vi "SolidTargetSequenceControl.vi"() -> ()   [LabVIEW 2015]
uses:
  ShootingStar/ShootingStar.lvlib
  State.ctl
  SolidTargetSequenceControl.lvlib
  <vilib>/Instr/_visa.llb/VISA Configure Serial Port (Instr).vi
  NetworkStream/NetworkStreamReceiverState.ctl
  NetworkStream/NetworkStream.lvlib
  NetworkStream/NetworkStreamData.ctl
  <vilib>/dex/Stream Element Allocation Mode.ctl
  NetworkStream/NetworkStreamReceiverMainQueueCluster.ctl
  NetworkStream/NetworkStreamStateMachineVariable.ctl
  NetworkStream/NetworkStreamReceiverStatusEventCluster.ctl
  ConsumerLoopVariable.ctl
  <vilib>/Utility/error.llb/Error Cluster From Error Code.vi
  <vilib>/ErrorRing/Error Ring.xnode
panel:
  in  "Arduino Serial Port":refnum<visa-resource-name>="COM3"
  in  "Phidget Voltage (V)":dbl=2.0 min=-10.0 max=10.0 step=0.1
  out "Device State":T1
  out "Session Hash":u64
  out "Network Stream State Indicator":T2
  in  "Shoot Once":bool
  in  "Target Radius (mm)":dbl=50.6
  in  "Shooting Pos. (mm)":dbl=5.0
  in  "Acquisition Time (ms)":dbl=100.0
  in  "Shot Spacing (mm)":dbl=0.1
  in  "Target Edge Pos. (mm)":dbl
  in  "Stop Rotation":bool
  in  "Start Rotation":bool
  in  "Clear Phidget":bool
  in  "Trig Cam":bool
  out "Arduino Message":string
  in  "Clear Serial Error":bool
  out "Phidget Error Cluster":errorcluster
  out "Cible":cluster{dbl, dbl}(knob)={0.0, 5.935711578539576} scale=0.0..360.0
  out "SP RotatingSpeed \n(deg/s)":dbl
  out "SP RotatingSpeed \n(rad/s)":dbl
  out "Serial error":errorcluster caption="Serial Error Out"
  in  "Calibrate":bool
  in  "ResetShotUntil":bool
  out "Shot until (°)":dbl
  out "Target position (°)":dbl
  in  "stop":bool
  # "Target Settings"
  # "Target Rotation"
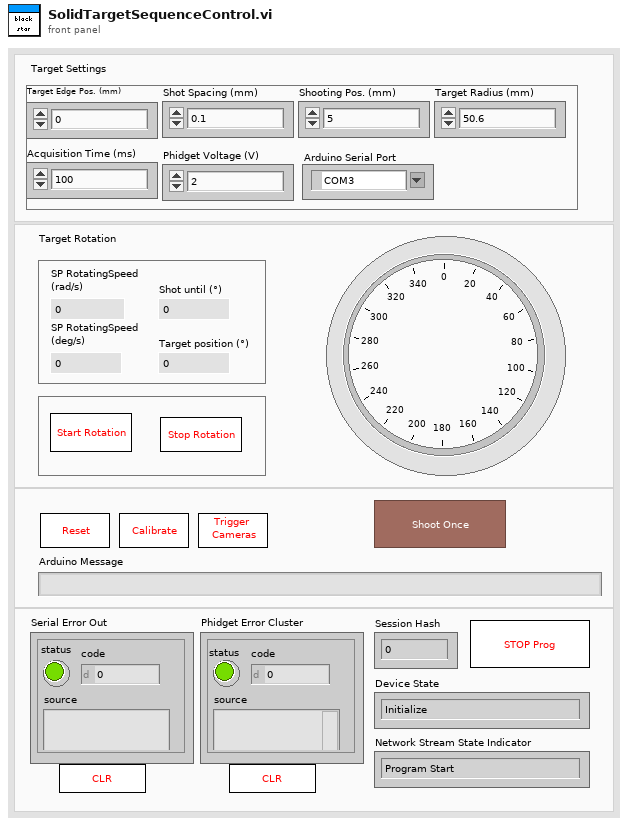
[diagram p1: front panel]
types:
  T1 = typedef "SolidTargetSequenceControl.lvlib/State.ctl" = enum16{"Initialize", "Running", "Closing"}
  T2 = typedef "NetworkStream.lvlib/NetworkStreamReceiverState.ctl" = enum16{"Program Start", "Waiting for connection", "Connected", "Connection lost", "Exit", "Unhandled Exception"}
  T3 = typedef "SolidTargetSequenceControl.lvlib/ConsumerLoopVariable.ctl" = cluster{"Arduino Serial Port":refnum<visa-resource-name>, "Phidget device handle":i32, "Arduino Message":string, "TargetRotating":bool}
  T4 = typedef "NetworkStream.lvlib/NetworkStreamReceiverStatusEventCluster.ctl" = cluster{"Status":string, "Data":variant, "SequenceNumber":u64}
  T5 = typedef "NetworkStream.lvlib/NetworkStreamStateMachineVariable.ctl" = cluster{"Network Stream Reader Endpoint":refnum<k21>, "Last Received Sequence Number":u64}
  T6 = typedef "NetworkStream.lvlib/NetworkStreamReceiverMainQueueCluster.ctl" = cluster{"Command":string, "Data":variant, "SequenceNumber":u64}
  T7 = enum8{"Enabled", "Disabled", "Disabled and Grayed Out"}
  T8 = typedef "NetworkStream.lvlib/NetworkStreamData.ctl" = cluster{"Command/Status":string, "Data":variant, "Session Hash":u64, "Sequence Number":u64}
  T9 = typedef "Stream Element Allocation Mode.ctl" = u32
  T10 = cluster{"Command/Status":string, "Data":variant, "Sequence Number":u64}
  T11 = cluster{"Status":string, "Data":variant, "Session Hash":u64, "SequenceNumberOfFinishedCommand":u64}
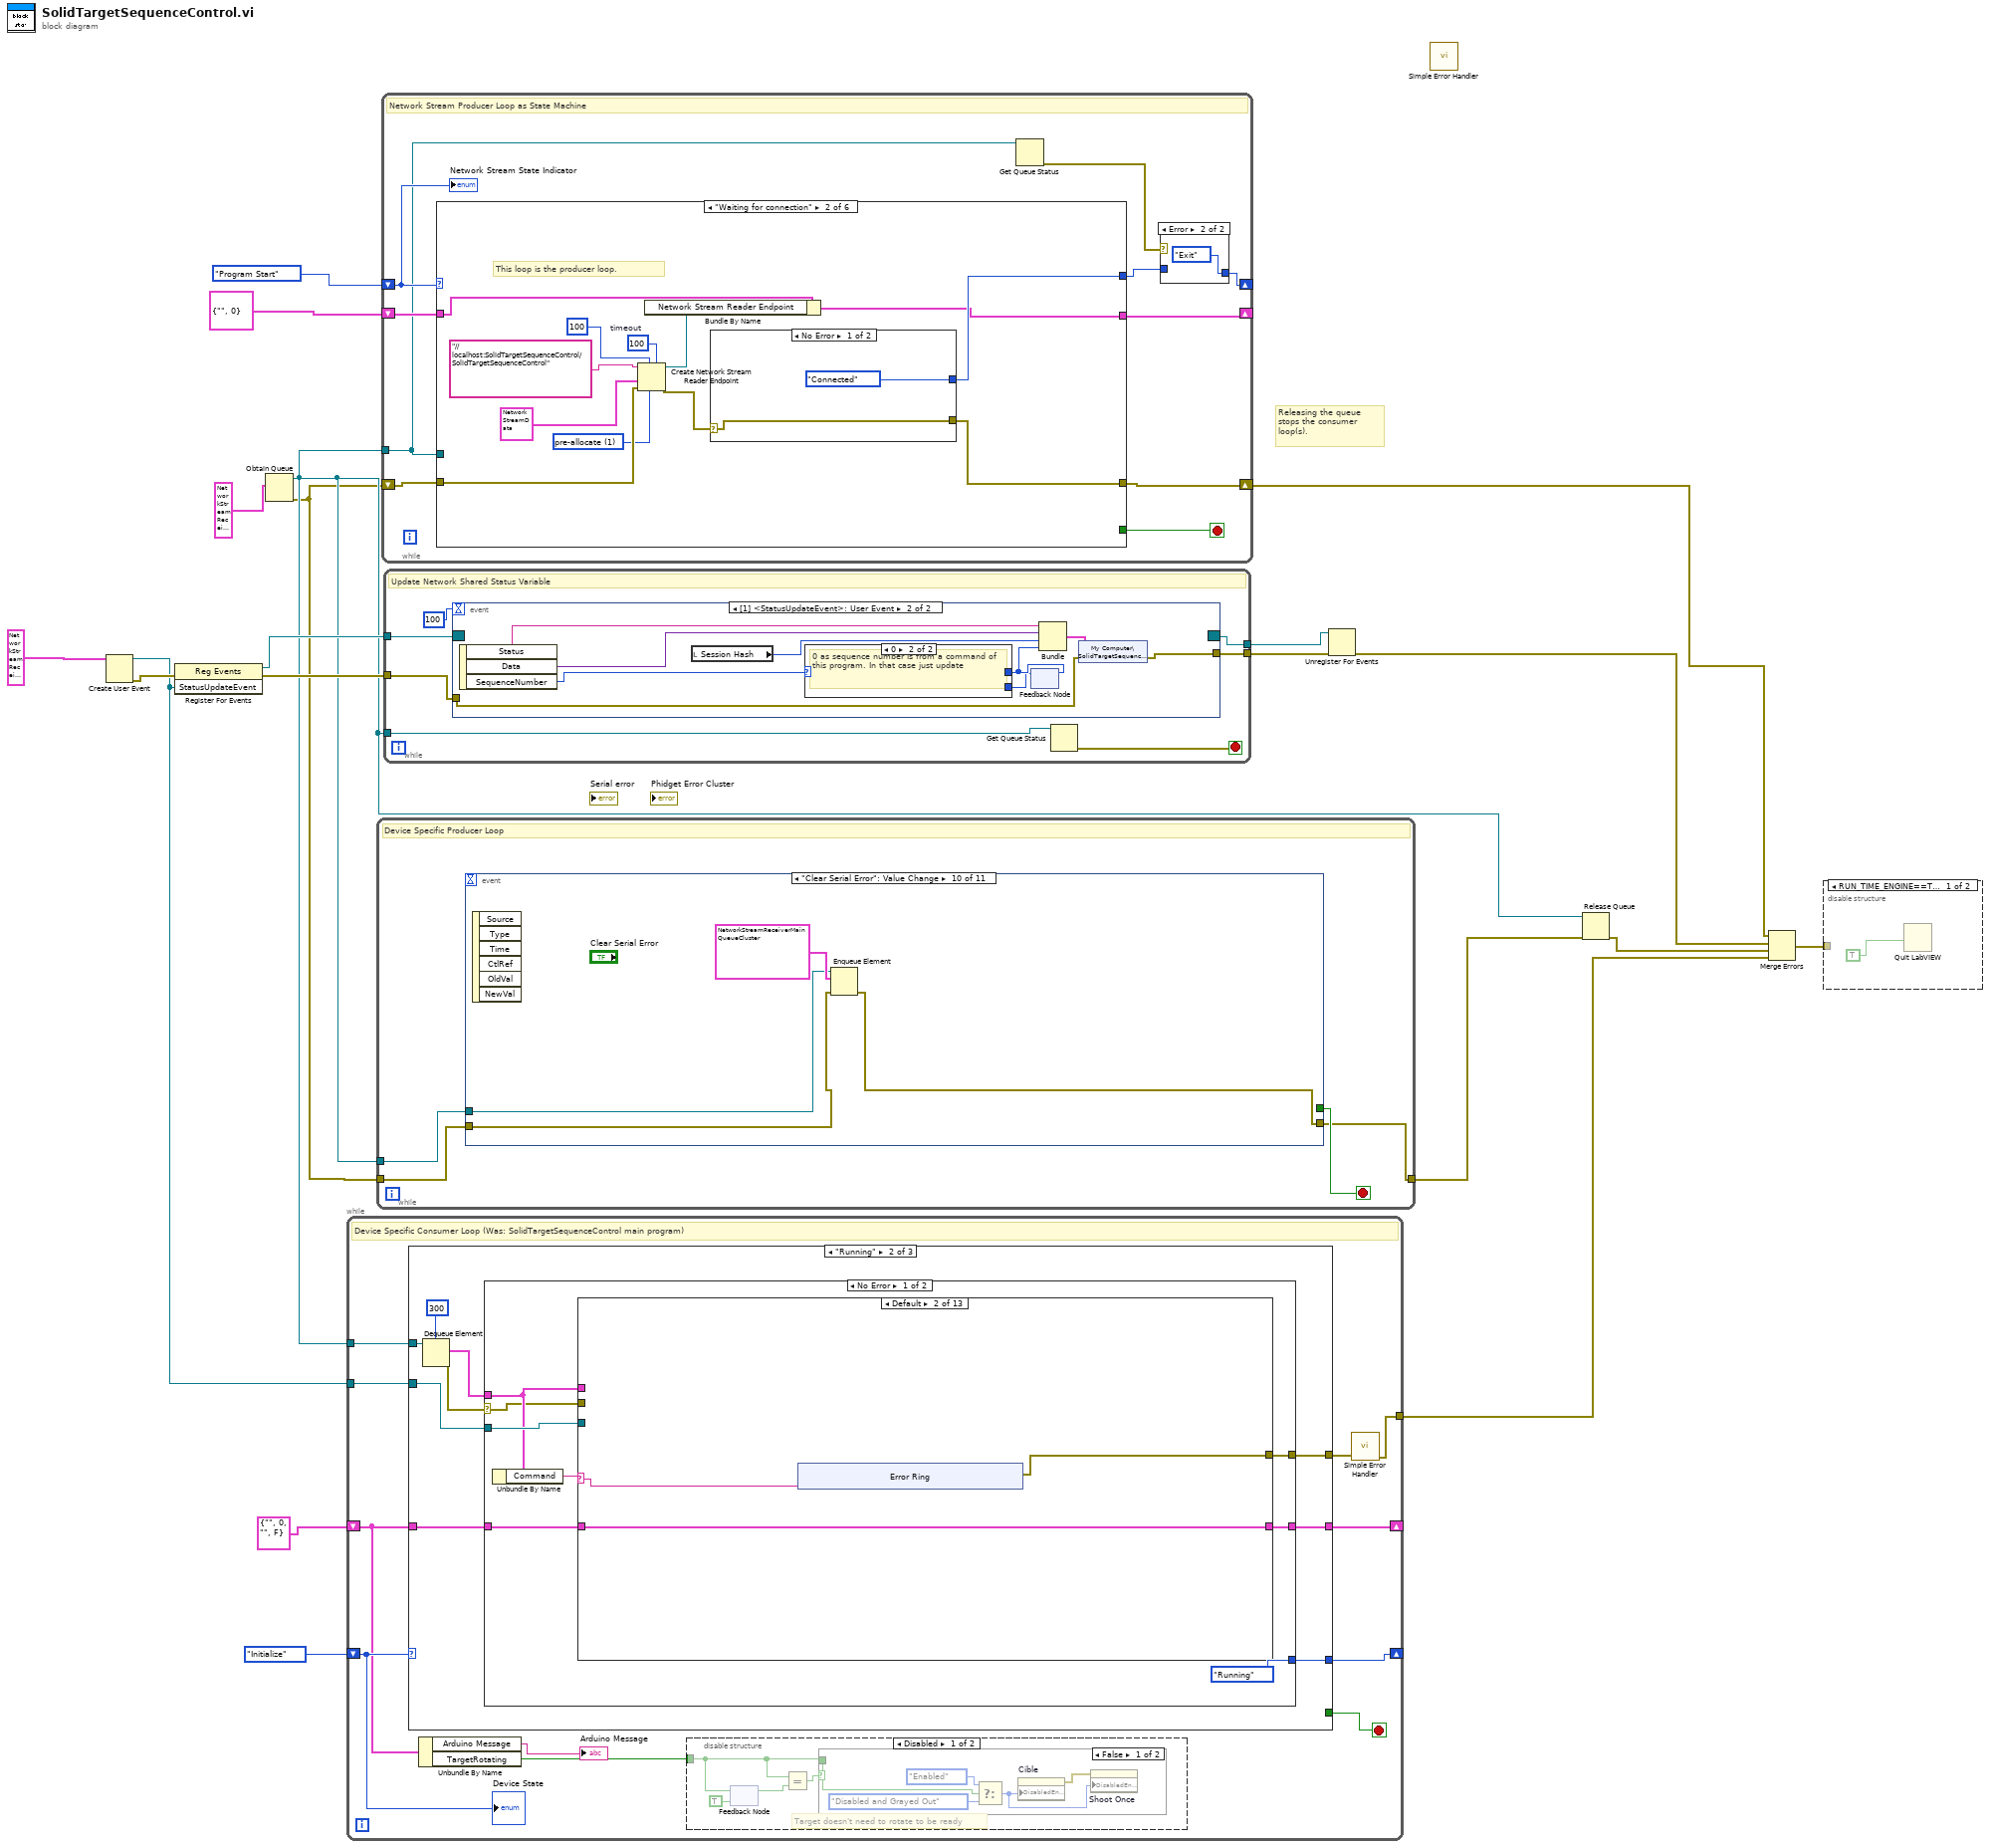
[diagram p0: block diagram]
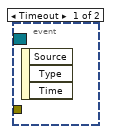
[diagram p2: hidden frame]
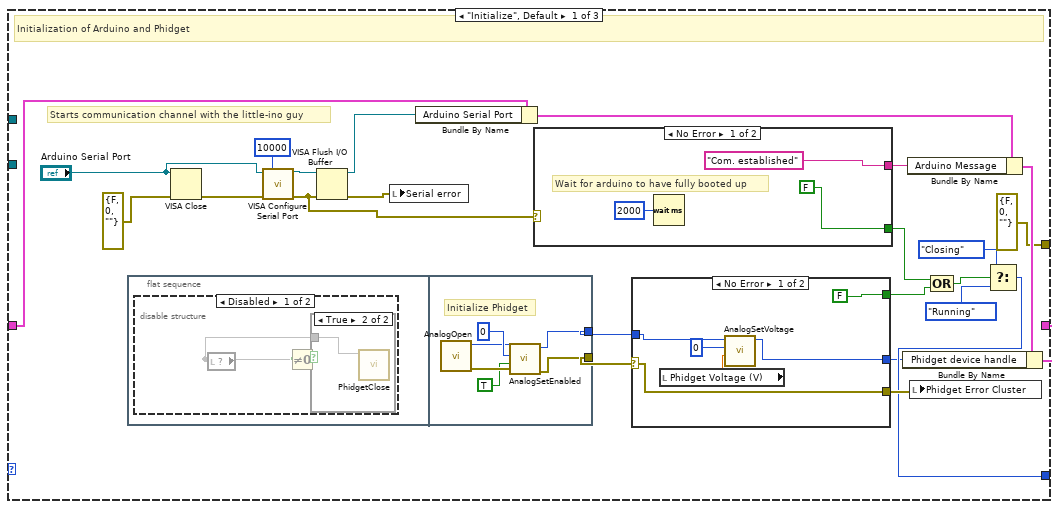
[diagram p6: hidden frame]
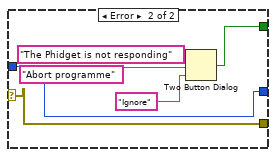
[diagram p7: hidden frame]
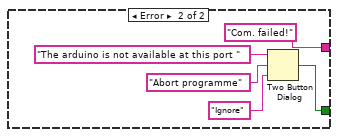
[diagram p10: hidden frame]
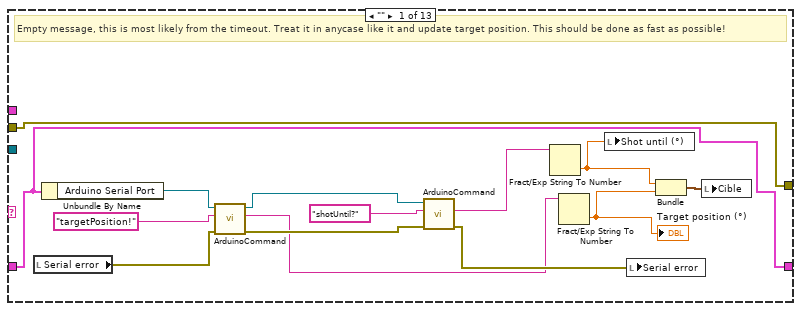
[diagram p11: hidden frame]
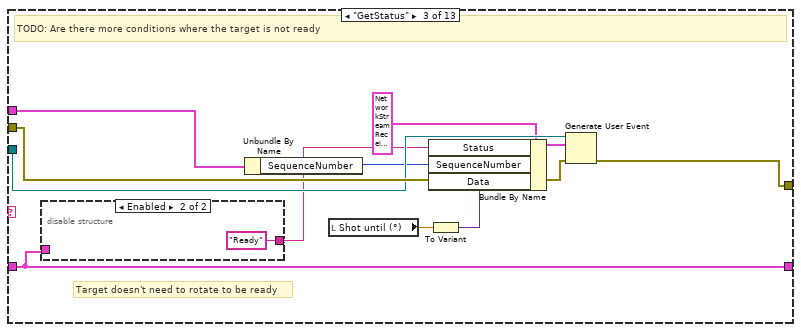
[diagram p12: hidden frame]
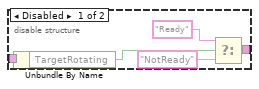
[diagram p13: hidden frame]
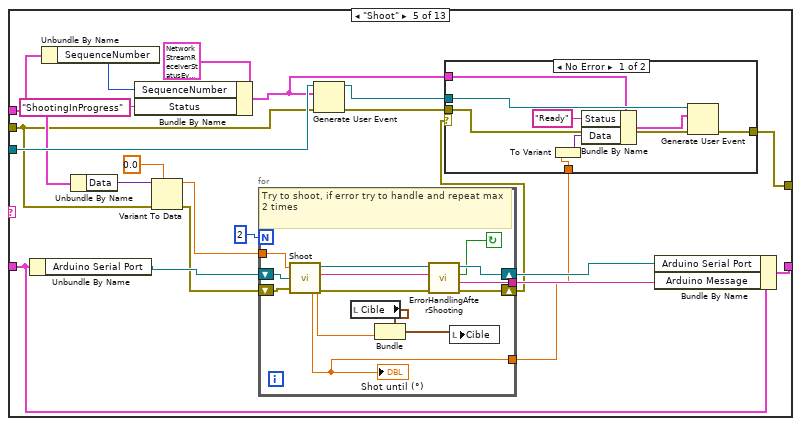
[diagram p15: hidden frame]
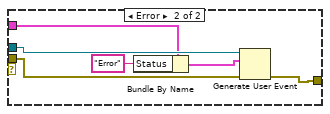
[diagram p16: hidden frame]
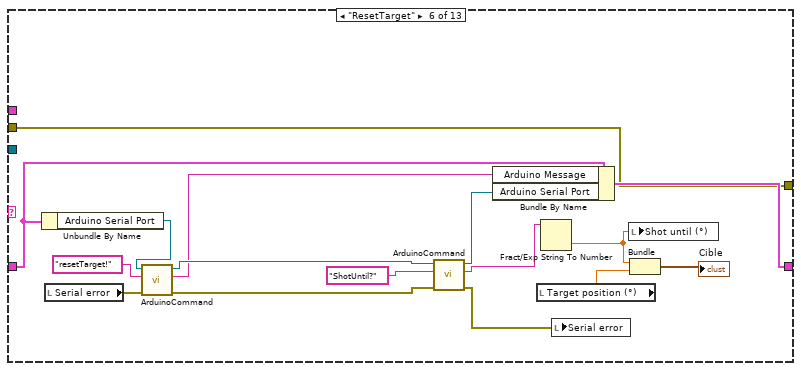
[diagram p17: hidden frame]
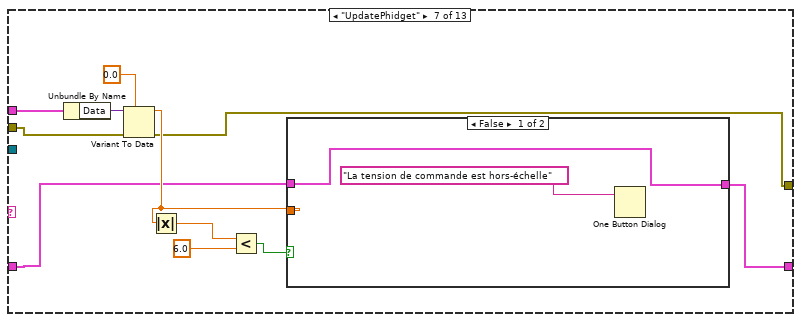
[diagram p18: hidden frame]
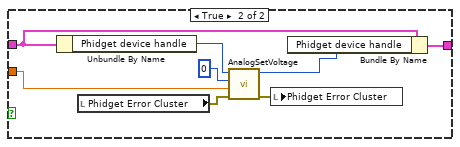
[diagram p19: hidden frame]
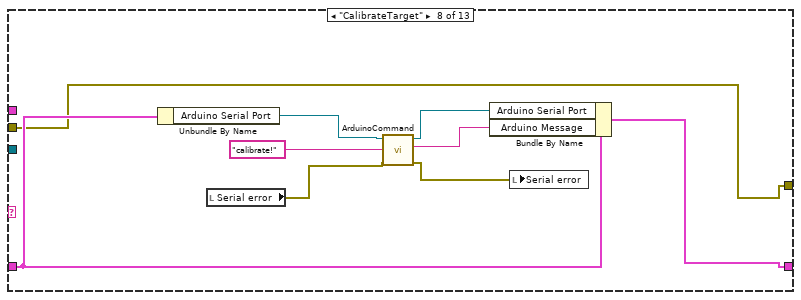
[diagram p20: hidden frame]
diagram:
  # "Releasing the queue stops the consumer loop(s)."
  n1 = Create User Event(user event datatype=T4 {"Status"="", "Data"=variant, "SequenceNumber"=0} ("StatusUpdateEvent")) -> (user event=w11:refnum<user-event>, error out=w17:errorcluster)  [unwired: 1 in]
  n2 = register-events(error in=w17, w11) -> (reference out=w16:refnum<event-registration>, error out=w13:errorcluster)  [unwired: 1 in]
  n3 = Obtain Queue(element data type=T6 {"Command"="", "Data"=variant, "SequenceNumber"=0}) -> (queue out=w10:refnum<queue>, error out=w9:errorcluster)  [unwired: 4 in, 1 out]
  n4 = while {
    tunnel: w10 -> [w31]
    tunnel: w11 -> [w29]
    tunnel: [w22] -> w3
    shift-right: [w27] -> _
    shift-left: State."Initialize" -> [w28]
    shift-right: [w26] -> _
    shift-left: T3 {"Arduino Serial Port"="", "Phidget device handle"=0, "Arduino Message"="", "TargetRotating"=FALSE} ("Cluster") -> [w24]
    stop <- w30 stop-if-true
    # "Device Specific Consumer Loop (Was: SolidTargetSequenceControl main program)"
    n5 = case shown="\"Running\"" w28 {
      tunnel: w31 -> [_ w102 _]
      tunnel: [_ _ TRUE] -> w30
      tunnel: w29 -> [_ w99 _]
      tunnel: [w50 w98 State."Initialize"] -> w27
      tunnel: w24 -> [w48 w96 w319]
      tunnel: [w45 w95 T3 {"Arduino Serial Port"="", "Phidget device handle"=0, "Arduino Message"="Connection Closed", "TargetRotating"=FALSE} ("Cluster")] -> w26
      tunnel: [errorcluster {"status"=FALSE, "code"=0, "source"=""} ("error out") w97 errorcluster {"status"=FALSE, "code"=0, "source"=""} ("error out")] -> w23
      frame "Initialize", Default {
        # "Starts communication channel with the little-ino guy"
        # "Initialization of Arduino and Phidget"
        n6 = flat-sequence {
          tunnel: [w81] -> w61
          tunnel: [w80] -> w62
          frame #0 {
            n7 = disable-structure shown="Disabled" {
              frame Disabled {
                n8 = local read item#-1() -> (w77)
                n9 = Not Equal To 0?(x=w77) -> (x != 0?=w78:bool)
                n10 = case shown="True" w78 {
                  tunnel: w77 -> [_ w79]
                  frame False {
                  }
                  frame True {
                    n11 = call "PhidgetClose.vi"("Device In"=w79) -> ()  [unwired: 10 in, 1 out]
                  }
                }
              }
              frame Enabled {
              }
            }
          }
          frame #1 {
            # "Initialize Phidget"
            n12 = call "AnalogOpen.vi"() -> ("error out"=w85:errorcluster, "Device Out"=w82:i32)  [unwired: 8 in, 2 out]
            n13 = call "AnalogSetEnabled.vi"("error in (no error)"=w85, "SetEnabled"=TRUE, "index"=0, "Device In"=w82) -> ("error out"=w80:errorcluster, "Device Out"=w81:i32)  [unwired: 5 in]
          }
        }
        n14 = VISA Close(VISA resource name="Arduino Serial Port", error in (no error)=errorcluster {"status"=FALSE, "code"=0, "source"=""}) -> (error out=w57:errorcluster)
        n15 = call-poly "VISA Configure Serial Port"("VISA resource name"="Arduino Serial Port", "timeout (10sec)"=u32 10000, "error in (no error)"=w57) -> ("VISA resource name out"=w58:refnum<visa-resource-name>, "error out"=w60:errorcluster)  [unwired: 11 in]
        n16 = VISA Flush I/O Buffer(VISA resource name=w58, error in (no error)=w60) -> (VISA resource name out=w47:refnum<visa-resource-name>, error out=w55:errorcluster)  [unwired: 1 in]
        n17 = local write "Serial error"(w55) -> ()
        n18 = Bundle By Name(cluster=w48, "Arduino Serial Port"=w47) -> (w44:T3)
        n19 = case shown="No Error" w60 {
          tunnel: [FALSE ("T button?") w92] -> w53
          tunnel: ["Com. established" ("Arduino Message") "Com. failed!" ("Arduino Message")] -> w42
          frame No Error {
            # "Wait for arduino to have fully booted up"
            n20 = Wait (ms)(milliseconds to wait=u32 2000) -> ()  [unwired: 1 out]
          }
          frame Error {
            n21 = Two Button Dialog(message="The arduino is not available at this port ", 1:"Ignore" ("Nom du bouton V (\"OK\")"), 2:"Abort programme" ("Nom du bouton V (\"OK\")")) -> (T button?=w92:bool)
          }
        }
        n22 = case shown="No Error" w62 {
          selector: w62 -> [w66 w72]
          tunnel: [FALSE w73] -> w54
          tunnel: w61 -> [w69 w71]
          tunnel: [w66 w72] -> w59
          tunnel: [w65 w71] -> w46
          frame No Error {
            n23 = local read "Phidget Voltage (V)"() -> (w67:dbl)
            n24 = call "AnalogSetVoltage.vi"("voltage"=w67, "index"=0, "Device In"=w69) -> ("Device Out"=w65:i32)  [unwired: 6 in, 1 out]
          }
          frame Error {
            n25 = Two Button Dialog(message="The Phidget is not responding", 1:"Ignore" ("Nom du bouton V (\"OK\")"), 2:"Abort programme" ("Nom du bouton V (\"OK\")")) -> (T button?=w73:bool)
          }
        }
        n26 = Bundle By Name(cluster=w44, "Arduino Message"=w42) -> (w43:T3)
        n27 = Bundle By Name(cluster=w43, "Phidget device handle"=w46) -> (w45:T3)
        n28 = local write "Phidget Error Cluster"(w59) -> ()
        n29 = Compound Arithmetic op=OR(w53, w54) -> (w52:bool)
        n30 = Select(t=State."Closing", s=w52, f=State."Running") -> (s? t:f=w50:T1)
      }
      frame "Running" {
        n31 = Dequeue Element(queue=w102, timeout in ms (-1)=300) -> (element=w100:T6, error out=w101:errorcluster)  [unwired: 1 in, 2 out]
        n32 = case shown="No Error" w101 {
          selector: w101 -> [w106 w313]
          tunnel: w100 -> [w108 _]
          tunnel: w99 -> [w110 _]
          tunnel: [State."Running" w314] -> w98
          tunnel: [w105 w312] -> w97
          tunnel: w96 -> [w104 w310]
          tunnel: [w103 w309] -> w95
          frame No Error {
            n33 = Unbundle By Name(w108) -> ("Command"=w109:string)
            n34 = case shown="Default" w109 {
              selector: w109 -> [_ w127 _ _ _ _ _ _ _ _ _ _ _]
              tunnel: w110 -> [_ _ w144 _ w175 _ _ _ _ _ _ _ _]
              tunnel: w108 -> [_ _ w141 _ w170 _ w226 _ _ _ _ _ _]
              tunnel: w106 -> [w111 _ w145 w152 w166 w204 w222 w242 w249 w260 w274 w280 w302]
              tunnel: [w111 w126 w139 w152 w156 w204 w221 w242 w249 w260 w274 w280 w302] -> w105
              tunnel: w104 -> [w112 w125 w138 w153 w163 w207 w220 w244 w254 w262 w276 w283 w304]
              tunnel: [w112 w125 w138 w153 w164 w205 w219 w243 w250 w261 w275 w281 w303] -> w103
              frame "" {
                # "Empty message, this is most likely from the timeout. Treat it in anycase like it and update target position. This should be done as fast as possible!"
                n35 = local read "Serial error"() -> (w118:errorcluster)
                n36 = Unbundle By Name(w112) -> ("Arduino Serial Port"=w113:refnum<visa-resource-name>)
                n37 = call "ArduinoCommand.vi"("entrée d'erreur (pas d'erreur)"=w118, "buffer à écrire"="targetPosition!", "Refnum VISA en entrée"=w113) -> ("sortie d'erreur"=w121:errorcluster, "read buffer"=w117:string, "Refnum VISA en sortie"=w119:refnum<visa-resource-name>)  [unwired: 6 in]
                n38 = call "ArduinoCommand.vi"("entrée d'erreur (pas d'erreur)"=w121, "buffer à écrire"="shotUntil?", "Refnum VISA en entrée"=w119) -> ("sortie d'erreur"=w122:errorcluster, "read buffer"=w123:string)  [unwired: 6 in, 1 out]
                n39 = Fract/Exp String To Number(string=w123) -> (number=w115:dbl)  [unwired: 3 in, 1 out]
                n40 = Fract/Exp String To Number(string=w117) -> (number=w124:dbl)  [unwired: 3 in, 1 out]
                "Target position (°)" <- w124
                n41 = local write "Shot until (°)"(w115) -> ()
                n42 = local write "Serial error"(w122) -> ()
                n43 = Bundle(w115, w124) -> (w114:cluster{dbl, dbl})  [unwired: 1 in]
                n44 = local write "Cible"(w114) -> ()
              }
              frame Default {
                n45 = xnode "Error Ring"("parameter 0"=w127) -> ("error out"=w126:errorcluster)
              }
              frame "GetStatus" {
                # "Target doesn't need to rotate to be ready"
                # "TODO: Are there more conditions where the target is not ready"
                n46 = disable-structure shown="Enabled" {
                  disable-tunnel: w138 -> [w150 _]
                  disable-tunnel: [w147 "Ready" ("f")] -> w137
                  frame Disabled {
                    n47 = Unbundle By Name(w150) -> ("TargetRotating"=w148:bool)
                    n48 = Select(t="Ready" ("Status"), s=w148, f="NotReady") -> (s? t:f=w147:string)
                  }
                  frame Enabled {
                  }
                }
                n49 = Unbundle By Name(w141) -> ("SequenceNumber"=w140:u64)
                n50 = local read "Shot until (°)"() -> (w135:dbl)
                n51 = To Variant(anything=w135) -> (Variant=w136:variant)
                n52 = Bundle By Name(cluster=T4 {"Status"="", "Data"=variant, "SequenceNumber"=0} ("event data"), "Status"=w137, "SequenceNumber"=w140, "Data"=w136) -> (w142:T4)
                n53 = Generate User Event(user event=w144, event data cluster=w142, error in=w145) -> (error out=w139:errorcluster)  [unwired: 1 in, 1 out]
              }
              frame "Reinitialize" {
                # "Todo: Implement"
              }
              frame "Shoot" {
                n54 = Unbundle By Name(w163) -> ("Arduino Serial Port"=w165:refnum<visa-resource-name>)
                n55 = Unbundle By Name(w170) -> ("SequenceNumber"=w173:u64)
                n56 = Unbundle By Name(w170) -> ("Data"=w169:variant)
                n57 = Bundle By Name(cluster=T4 {"Status"="", "Data"=variant, "SequenceNumber"=0} ("StatusUpdateEvent"), "SequenceNumber"=w173, "Status"="ShootingInProgress") -> (w155:T4)
                n58 = Variant To Data(error in=w166, type=0.0 ("Acquisition Time (ms) 2"), Variant=w169) -> (data=w167:dbl, error out=w160:errorcluster)
                n59 = for {
                  N: 2 -> [_]
                  tunnel: [w195] -> w161
                  tunnel: w167 -> [w194]
                  shift-right: [w197] -> w162
                  shift-left: w165 -> [w202]
                  shift-right: [w199] -> w159
                  shift-left: w160 -> [w201]
                  tunnel: [w190] -> w154
                  stop <- w191 continue-if-true
                  # "Try to shoot, if error try to handle and repeat max 2 times"
                  n60 = call "Shoot.vi"("Shoot during x ms"=w194, "Arduino Serial Port"=w202, "error in (no error)"=w201) -> ("Arduino Serial out"=w198:refnum<visa-resource-name>, "Message"=w196:string, "Shot Unitil"=w190:dbl, "error out"=w200:errorcluster)
                  "Shot until (°)" <- w190
                  n61 = local read "Cible"() -> (w192:cluster{dbl, dbl})
                  n62 = Bundle(cluster=w192, w190) -> (w193:cluster{dbl, dbl})  [unwired: 1 in]
                  n63 = call "ErrorHandlingAfterShooting.vi"("error in (no error)"=w200, "Arduino Message IN"=w196, "Nom de ressource VISA IN"=w198) -> ("error out"=w199:errorcluster, "Arduino Message OUT"=w195:string, "Try Shooting Again"=w191:bool, "Nom de ressource VISA OUT"=w197:refnum<visa-resource-name>)  [unwired: 3 in]
                  n64 = local write "Cible"(w193) -> ()
                }
                n65 = Generate User Event(user event=w175, event data cluster=w155, error in=w166) -> (user event out=w158:refnum<user-event>, error out=w157:errorcluster)  [unwired: 1 in]
                n66 = case shown="No Error" w159 {
                  tunnel: w158 -> [w183 w186]
                  tunnel: w157 -> [w182 w184]
                  tunnel: [w181 w187] -> w156
                  tunnel: w155 -> [w179 w185]
                  tunnel: w154 -> [w177 _]
                  frame No Error {
                    n67 = To Variant(anything=w177) -> (Variant=w176:variant)
                    n68 = Bundle By Name(cluster=w179, "Status"="Ready", "Data"=w176) -> (w180:T4)
                    n69 = Generate User Event(user event=w183, event data cluster=w180, error in=w182) -> (error out=w181:errorcluster)  [unwired: 1 in, 1 out]
                  }
                  frame Error {
                    n70 = Bundle By Name(cluster=w185, "Status"="Error") -> (w188:T4)
                    n71 = Generate User Event(user event=w186, event data cluster=w188, error in=w184) -> (error out=w187:errorcluster)  [unwired: 1 in, 1 out]
                  }
                }
                n72 = Bundle By Name(cluster=w163, "Arduino Serial Port"=w162, "Arduino Message"=w161) -> (w164:T3)
              }
              frame "ResetTarget" {
                n73 = Unbundle By Name(w207) -> ("Arduino Serial Port"=w208:refnum<visa-resource-name>)
                n74 = local read "Serial error"() -> (w212:errorcluster)
                n75 = call "ArduinoCommand.vi"("entrée d'erreur (pas d'erreur)"=w212, "buffer à écrire"="resetTarget!", "Refnum VISA en entrée"=w208) -> ("sortie d'erreur"=w215:errorcluster, "read buffer"=w203:string, "Refnum VISA en sortie"=w213:refnum<visa-resource-name>)  [unwired: 6 in]
                n76 = call "ArduinoCommand.vi"("entrée d'erreur (pas d'erreur)"=w215, "buffer à écrire"="ShotUntil?", "Refnum VISA en entrée"=w213) -> ("sortie d'erreur"=w216:errorcluster, "read buffer"=w217:string, "Refnum VISA en sortie"=w206:refnum<visa-resource-name>)  [unwired: 6 in]
                n77 = Bundle By Name(cluster=w207, "Arduino Message"=w203, "Arduino Serial Port"=w206) -> (w205:T3)
                n78 = local read "Target position (°)"() -> (w210:dbl)
                n79 = Fract/Exp String To Number(string=w217) -> (number=w209:dbl)  [unwired: 3 in, 1 out]
                n80 = local write "Serial error"(w216) -> ()
                n81 = local write "Shot until (°)"(w209) -> ()
                n82 = Bundle(w209, "Target position (°)"=w210) -> (→"Cible":cluster{dbl, "Target position (°)":dbl})  [unwired: 1 in]
              }
              frame "UpdatePhidget" {
                n83 = Unbundle By Name(w226) -> ("Data"=w225:variant)
                n84 = Variant To Data(error in=w222, type=0.0 ("Phidget Voltage (V) 2"), Variant=w225) -> (data=w223:dbl, error out=w221:errorcluster)
                n85 = Absolute Value(x=w223) -> (abs(x)=w227:dbl)
                n86 = Less?(x=w227, y=6.0) -> (x < y?=w229:bool)
                n87 = case shown="False" w229 {
                  tunnel: w223 -> [_ w236]
                  tunnel: w220 -> [w230 w233]
                  tunnel: [w230 w232] -> w219
                  frame False {
                    n88 = One Button Dialog(message="La tension de commande est hors-échelle") -> ()  [unwired: 1 in, 1 out]
                  }
                  frame True {
                    n89 = Unbundle By Name(w233) -> ("Phidget device handle"=w234:i32)
                    n90 = local read "Phidget Error Cluster"() -> (w237:errorcluster)
                    n91 = call "AnalogSetVoltage.vi"("error in (no error)"=w237, "voltage"=w236, "index"=0, "Device In"=w234) -> ("error out"=w238:errorcluster, "Device Out"=w235:i32)  [unwired: 5 in]
                    n92 = local write "Phidget Error Cluster"(w238) -> ()
                    n93 = Bundle By Name(cluster=w233, "Phidget device handle"=w235) -> (w232:T3)
                  }
                }
              }
              frame "CalibrateTarget" {
                n94 = Unbundle By Name(w244) -> ("Arduino Serial Port"=w245:refnum<visa-resource-name>)
                n95 = local read "Serial error"() -> (w247:errorcluster)
                n96 = call "ArduinoCommand.vi"("entrée d'erreur (pas d'erreur)"=w247, "buffer à écrire"="calibrate!", "Refnum VISA en entrée"=w245) -> ("sortie d'erreur"=w248:errorcluster, "read buffer"=w241:string, "Refnum VISA en sortie"=w240:refnum<visa-resource-name>)  [unwired: 6 in]
                n97 = Bundle By Name(cluster=w244, "Arduino Serial Port"=w240, "Arduino Message"=w241) -> (w243:T3)
                n98 = local write "Serial error"(w248) -> ()
              }
              frame "TriggerCameras" {
                n99 = Unbundle By Name(w254) -> ("Arduino Serial Port"=w253:refnum<visa-resource-name>)
                n100 = local read "Serial error"() -> (w256:errorcluster)
                n101 = call "ArduinoCommand.vi"("entrée d'erreur (pas d'erreur)"=w256, "buffer à écrire"="triggerCameras!", "Refnum VISA en entrée"=w253) -> ("sortie d'erreur"=w257:errorcluster, "read buffer"=w251:string, "Refnum VISA en sortie"=w252:refnum<visa-resource-name>)  [unwired: 6 in]
                n102 = local write "Serial error"(w257) -> ()
                n103 = Bundle By Name(cluster=w254, "Arduino Serial Port"=w252, "Arduino Message"=w251) -> (w250:T3)
              }
              frame "StartTargetMotor" {
                n104 = Unbundle By Name(w262) -> ("Arduino Serial Port"=w263:refnum<visa-resource-name>)
                n105 = local read "Serial error"() -> (w266:errorcluster)
                n106 = call "ArduinoCommand.vi"("entrée d'erreur (pas d'erreur)"=w266, "buffer à écrire"="startMotor!", "Refnum VISA en entrée"=w263) -> ("sortie d'erreur"=w267:errorcluster, "read buffer"=w259:string, "Refnum VISA en sortie"=w264:refnum<visa-resource-name>)  [unwired: 6 in]
                n107 = local write "Serial error"(w267) -> ()
                n108 = case shown="\"ok\\r\\n\"" w259 {
                  tunnel: [FALSE ("TargetRotating") TRUE ("TargetRotating")] -> w258
                  frame "False", Default {
                  }
                  frame "ok\r\n" {
                  }
                }
                n109 = Bundle By Name(cluster=w262, "TargetRotating"=w258, "Arduino Serial Port"=w264, "Arduino Message"=w259) -> (w261:T3)
              }
              frame "StopTargetMotor" {
                n110 = Unbundle By Name(w276) -> ("Arduino Serial Port"=w273:refnum<visa-resource-name>)
                n111 = local read "Serial error"() -> (w278:errorcluster)
                n112 = call "ArduinoCommand.vi"("entrée d'erreur (pas d'erreur)"=w278, "buffer à écrire"="stopMotor!", "Refnum VISA en entrée"=w273) -> ("sortie d'erreur"=w279:errorcluster, "read buffer"=w272:string, "Refnum VISA en sortie"=w271:refnum<visa-resource-name>)  [unwired: 6 in]
                n113 = Bundle By Name(cluster=w276, "TargetRotating"=FALSE, "Arduino Serial Port"=w271, "Arduino Message"=w272) -> (w275:T3)
                n114 = local write "Serial error"(w279) -> ()
              }
              frame "ClearPhidgetError" {
                n115 = Unbundle By Name(w283) -> ("Phidget device handle"=w284:i32)
                n116 = local read "Phidget Error Cluster"() -> (w286:errorcluster)
                n117 = call "PhidgetClose.vi"("error in"=w286, "Device In"=w284) -> ("error out"=w285:errorcluster)  [unwired: 9 in]
                n118 = call "ErrorHandler.vi"("error in"=w285) -> ("error out"=w287:errorcluster)  [unwired: 9 in, 1 out]
                n119 = case shown="Error" w287 {
                  selector: w287 -> [w289 w301]
                  tunnel: [w288 0 ("Device Out")] -> w282
                  frame No Error {
                    n120 = local read "Phidget Voltage (V)"() -> (w292:dbl)
                    n121 = call "PhidgetOpen.vi"("error in"=w289, "Device In"=i64 0) -> ("error out"=w296:errorcluster, "Device Out"=w297:i32)  [unwired: 6 in, 2 out]
                    n122 = call "AnalogSetEnabled.vi"("error in (no error)"=w296, "SetEnabled"=TRUE, "index"=0, "Device In"=w297) -> ("error out"=w293:errorcluster, "Device Out"=w294:i32)  [unwired: 5 in]
                    n123 = call "AnalogSetVoltage.vi"("error in (no error)"=w293, "voltage"=w292, "index"=0, "Device In"=w294) -> ("error out"=w290:errorcluster, "Device Out"=w288:i32)  [unwired: 5 in]
                    n124 = local write "Phidget Error Cluster"(w290) -> ()
                  }
                  frame Error {
                    n125 = local write "Phidget Error Cluster"(w301) -> ()
                  }
                }
                n126 = Bundle By Name(cluster=w283, "Phidget device handle"=w282) -> (w281:T3)
              }
              frame "ClearArduinoError" {
                n127 = Unbundle By Name(w304) -> ("Arduino Serial Port"=w305:refnum<visa-resource-name>)
                n128 = VISA Flush I/O Buffer(VISA resource name=w305, error in (no error)=errorcluster {"status"=FALSE, "code"=0, "source"=""} ("Serial error")) -> (VISA resource name out=w306:refnum<visa-resource-name>, error out=w308:errorcluster)  [unwired: 1 in]
                n129 = Bundle By Name(cluster=w304, "Arduino Serial Port"=w306) -> (w303:T3)
                n130 = local write "Serial error"(w308) -> ()
              }
            }
          }
          frame Error {
            n131 = Unbundle By Name(w313) -> ("code"=w311:i32)
            n132 = case shown="1122, Default" w311 {
              tunnel: [State."Closing"] -> w314
              tunnel: [errorcluster {"status"=FALSE, "code"=0, "source"=""} ("error out")] -> w312
              tunnel: w310 -> [w315]
              tunnel: [w315] -> w309
              frame 1122, Default {
                # "Either the queue got terminated (Error code 1122), or another error occured. In any case exit the consumer loop"
              }
            }
          }
        }
      }
      frame "Closing" {
        # "Close Phidget"
        # "Close Arduino Connection"
        n133 = Unbundle By Name(w319) -> ("Arduino Serial Port"=w324:refnum<visa-resource-name>)
        n134 = Unbundle By Name(w319) -> ("Phidget device handle"=w320:i32)
        n135 = local read "Phidget Error Cluster"() -> (w323:errorcluster)
        n136 = VISA Close(VISA resource name=w324) -> (error out=w328:errorcluster)  [unwired: 1 in]
        n137 = call "PhidgetClose.vi"("error in"=w323, "Device In"=w320) -> ("error out"=w322:errorcluster)  [unwired: 9 in]
        n138 = local write "Serial error"(w328) -> ()
        n139 = call "ErrorHandler.vi"("error in"=w322) -> ("error out"=w321:errorcluster)  [unwired: 9 in, 1 out]
        n140 = local write "Phidget Error Cluster"(w321) -> ()
      }
    }
    n141 = Unbundle By Name(w24) -> ("Arduino Message"=→"Arduino Message":string, "TargetRotating"=w21:bool)
    n142 = disable-structure shown="Disabled" {
      disable-tunnel: w21 -> [w33 _]
      frame Disabled {
        # "Target doesn't need to rotate to be ready"
        n143 = feedback #1(TRUE ("TargetRotating")) -> (w32:bool)
        n144 = feedback-in #1(w33) -> ()
        n145 = Equal?(x=w33, y=w32) -> (x = y?=w34:bool)
        n146 = case shown="False" w34 {
          tunnel: w33 -> [w38 _]
          frame False {
            n147 = Select(t=T7."Enabled" ("Disabled"), s=w38, f=T7."Disabled and Grayed Out" ("Disabled")) -> (s? t:f=w36:T7)
            n148 = property on="Cible" class="Knob (strict)"("DisabledEnum"=w36) -> (error out=w37:errorcluster)  [unwired: 2 in, 1 out]
            n149 = property on="Shoot Once" class="Bool"(error in=w37, "DisabledEnum"=w36) -> ()  [unwired: 1 in, 2 out]
          }
          frame True {
          }
        }
      }
      frame Enabled {
      }
    }
    n150 = call <vilib>:"Simple Error Handler.vi"("error in (no error)"=w23) -> ("error out"=w22:errorcluster)  [unwired: 4 in, 4 out]
    "Device State" <- w28
  }
  n151 = while {
    tunnel: w10 -> [w331]
    tunnel: w9 -> [w330]
    tunnel: [w329] -> w8
    stop <- w332 stop-if-true
    # "Device Specific Producer Loop"
    n152 = event shown="[9] \"Clear Serial Error\": Value Change" {
      selector: _ -> [_ _ _ _ _ _ _ _ _ _ _]
      dyn-events: _ -> [_ _ _ _ _ _ _ _ _ _ _]
      timeout: _ -> [_ _ _ _ _ _ _ _ _ _ _]
      tunnel: [_ _ _ _ _ _ _ _ _ _ "stop"] -> w332
      tunnel: w331 -> [w333 w349 w354 w360 w368 w371 w375 w379 w383 w387 _]
      tunnel: w330 -> [w336 w348 w353 w359 w363 w370 w374 w378 w382 w386 w389]
      tunnel: [w334 w347 w352 w358 w362 w369 w373 w377 w381 w385 w389] -> w329
      event "Shooting Pos. (mm)", "Target Edge Pos. (mm)", "Shot Spacing (mm)", "Acquisition Time (ms)", "Target Radius (mm)": Value Change {
        n153 = event-data() -> ()  [unwired: 1 in, 6 out]
        n154 = call "CalculateTargetSpeed.vi"("Target Edge Pos. (mm)"="Target Edge Pos. (mm)", "Shooting Pos. (mm)"="Shooting Pos. (mm)", "Target Radius (mm)"="Target Radius (mm)", "Shot Spacing (mm)"="Shot Spacing (mm)") -> ("Numeric Control 2"=→"SP RotatingSpeed \n(deg/s)":dbl, "Numeric Control 3"=→"SP RotatingSpeed \n(rad/s)":dbl, "Numeric Control"=w337:dbl)  [unwired: 5 in]
        n155 = property on="Phidget Voltage (V)" class="DigNum (strict)"(error in=w336, "Value"=w337) -> (error out=w335:errorcluster)  [unwired: 1 in, 1 out]
        n156 = To Variant(anything=w337) -> (Variant=w338:variant)
        n157 = Bundle By Name(cluster=T6 {"Command"="UpdatePhidget", "Data"=variant, "SequenceNumber"=0} ("element"), "Data"=w338) -> (w339:T6)
        n158 = Enqueue Element(queue=w333, element=w339, error in (no error)=w335) -> (error out=w334:errorcluster)  [unwired: 1 in, 2 out]
      }
      event "ResetShotUntil": Value Change {
        n159 = event-data() -> ()  [unwired: 1 in, 6 out]
        n160 = Enqueue Element(queue=w349, element=T6 {"Command"="ResetTarget", "Data"=variant, "SequenceNumber"=0}, error in (no error)=w348) -> (error out=w347:errorcluster)  [unwired: 1 in, 2 out]
      }
      event "Phidget Voltage (V)": Value Change {
        n161 = event-data() -> ()  [unwired: 1 in, 6 out]
        n162 = To Variant(anything="Phidget Voltage (V)") -> (Variant=w355:variant)
        n163 = Bundle By Name(cluster=T6 {"Command"="UpdatePhidget", "Data"=variant, "SequenceNumber"=0} ("element"), "Data"=w355) -> (w356:T6)
        n164 = Enqueue Element(queue=w354, element=w356, error in (no error)=w353) -> (error out=w352:errorcluster)  [unwired: 1 in, 2 out]
      }
      event "Calibrate": Value Change {
        n165 = event-data() -> ()  [unwired: 1 in, 6 out]
        n166 = Enqueue Element(queue=w360, element=T6 {"Command"="CalibrateTarget", "Data"=variant, "SequenceNumber"=0}, error in (no error)=w359) -> (error out=w358:errorcluster)  [unwired: 1 in, 2 out]
      }
      event "Shoot Once": Value Change {
        n167 = event-data() -> ()  [unwired: 1 in, 6 out]
        n168 = To Variant(anything="Acquisition Time (ms)") -> (Variant=w364:variant)
        n169 = Bundle By Name(cluster=T6 {"Command"="Shoot", "Data"=variant, "SequenceNumber"=0} ("element"), "Data"=w364) -> (w366:T6)
        n170 = Enqueue Element(queue=w368, element=w366, error in (no error)=w363) -> (error out=w362:errorcluster)  [unwired: 1 in, 2 out]
      }
      event "Trig Cam": Value Change {
        n171 = event-data() -> ()  [unwired: 1 in, 6 out]
        n172 = Enqueue Element(queue=w371, element=T6 {"Command"="TriggerCameras", "Data"=variant, "SequenceNumber"=0}, error in (no error)=w370) -> (error out=w369:errorcluster)  [unwired: 1 in, 2 out]
      }
      event "Start Rotation": Value Change {
        n173 = event-data() -> ()  [unwired: 1 in, 6 out]
        n174 = Enqueue Element(queue=w375, element=T6 {"Command"="StartTargetMotor", "Data"=variant, "SequenceNumber"=0}, error in (no error)=w374) -> (error out=w373:errorcluster)  [unwired: 1 in, 2 out]
      }
      event "Stop Rotation": Value Change {
        n175 = event-data() -> ()  [unwired: 1 in, 6 out]
        n176 = Enqueue Element(queue=w379, element=T6 {"Command"="StopTargetMotor", "Data"=variant, "SequenceNumber"=0}, error in (no error)=w378) -> (error out=w377:errorcluster)  [unwired: 1 in, 2 out]
      }
      event "Clear Phidget": Value Change {
        n177 = event-data() -> ()  [unwired: 1 in, 6 out]
        n178 = Enqueue Element(queue=w383, element=T6 {"Command"="ClearPhidgetError", "Data"=variant, "SequenceNumber"=0}, error in (no error)=w382) -> (error out=w381:errorcluster)  [unwired: 1 in, 2 out]
      }
      event "Clear Serial Error": Value Change {
        n179 = event-data() -> ()  [unwired: 1 in, 6 out]
        n180 = Enqueue Element(queue=w387, element=T6 {"Command"="ClearPhidgetError", "Data"=variant, "SequenceNumber"=0}, error in (no error)=w386) -> (error out=w385:errorcluster)  [unwired: 1 in, 2 out]
      }
      event "stop": Value Change {
        n181 = event-data() -> ()  [unwired: 1 in, 6 out]
      }
    }
  }
  n182 = while {
    shift-right: [w393] -> w6
    shift-left: w9 -> [w394]
    shift-right: [w398] -> _
    shift-left: T5 {"Network Stream Reader Endpoint"="", "Last Received Sequence Number"=0} ("StateMachineVariable") -> [w399]
    shift-right: [w396] -> _
    shift-left: NetworkStreamReceiverState."Program Start" -> [w400]
    tunnel: w10 -> [w392]
    stop <- w395 stop-if-true
    # "This loop is the producer loop."
    # "Network Stream Producer Loop as State Machine"
    n183 = case shown="\"Waiting for connection\"" w400 {
      tunnel: [NetworkStreamReceiverState."Waiting for connection" w412 w433 NetworkStreamReceiverState."Waiting for connection" NetworkStreamReceiverState."Exit" NetworkStreamReceiverState."Exit"] -> w397
      tunnel: w394 -> [w404 w414 w437 w475 w484 w492]
      tunnel: [w404 w411 w434 w467 w483 w491] -> w393
      tunnel: w399 -> [w403 w410 w432 w472 w481 w490]
      tunnel: [w403 w408 w431 w470 w482 w490] -> w398
      tunnel: [_ _ _ _ TRUE _] -> w395
      tunnel: w392 -> [_ _ w430 _ _ _]
      frame "Program Start", Default {
      }
      frame "Waiting for connection" {
        w407 = T9 1 items=["allocate as needed", "pre-allocate"] ("element allocation mode")
        w417 = 100  # timeout
        n184 = Create Network Stream Reader Endpoint(5:w417, 6:w407, 7:100 ("reader buffer size"), 8:w414, 9:T8 {"Command/Status"="", "Data"=variant, "Session Hash"=0, "Sequence Number"=0} ("NetworkStreamCluster"), 11:"//localhost:SolidTargetSequenceControl/SolidTargetSequenceControl" ("reader name")) -> (0:w413:errorcluster, 3:w409:refnum<k21>)  [unwired: 1 in]
        n185 = Bundle By Name(cluster=w410, "Network Stream Reader Endpoint"=w409) -> (w408:T5)
        n186 = case shown="No Error" w413 {
          selector: w413 -> [w418 w421]
          tunnel: [NetworkStreamReceiverState."Connected" w423] -> w412
          tunnel: [w418 w420] -> w411
          frame No Error {
          }
          frame Error {
            n187 = Unbundle By Name(w421) -> ("code"=w422:i32)
            n188 = case shown="-314004" w422 {
              tunnel: [NetworkStreamReceiverState."Unhandled Exception" NetworkStreamReceiverState."Waiting for connection"] -> w423
              tunnel: w421 -> [w424 w427]
              tunnel: [w424 w426] -> w420
              frame 0, Default {
              }
              frame -314004 {
                # "Timed out, try again..."
                n189 = call <vilib>:"Clear Errors.vi"("error in (no error)"=w427, "specific error code to clear (0: all)"=-314004) -> ("error out"=w426:errorcluster)  [unwired: 4 in, 1 out]
              }
            }
          }
        }
      }
      frame "Connected" {
        n190 = Unbundle By Name(w432) -> ("Network Stream Reader Endpoint"=w436:refnum<k21>)
        n191 = shared-variable-read "Read Single Element from Stream"(w436, w437, 100 ("timeout ms (-1)")) -> (w435:errorcluster, w439:bool, w438:T8)  [unwired: 1 out]
        n192 = case shown="No Error" w435 {
          selector: w435 -> [w446 w463]
          tunnel: w439 -> [w448 _]
          tunnel: w438 -> [w447 _]
          tunnel: [w445 w463] -> w434
          tunnel: [NetworkStreamReceiverState."Connected" w461] -> w433
          tunnel: w432 -> [w443 w464]
          tunnel: [w442 w464] -> w431
          tunnel: w430 -> [w441 _]
          frame No Error {
            n193 = case shown="False" w448 {
              tunnel: [w455 w460] -> w445
              tunnel: w446 -> [w456 w460]
              tunnel: w447 -> [w458 _]
              tunnel: w443 -> [w449 w459]
              tunnel: [w449 w459] -> w442
              tunnel: w441 -> [w457 _]
              frame False {
                n194 = Unbundle By Name(w458) -> ("Session Hash"=→"Session Hash":u64, "Sequence Number"=w451:u64, "Command/Status"=w454:string, "Data"=w453:variant)
                n195 = Bundle("Command/Status"=w454, "Data"=w453, "Sequence Number"=w451) -> (w452:T10)  [unwired: 1 in]
                n196 = Enqueue Element(queue=w457, element=w452, error in (no error)=w456) -> (error out=w455:errorcluster)  [unwired: 1 in, 2 out]
              }
              frame True {
              }
            }
          }
          frame Error {
            n197 = Unbundle By Name(w463) -> ("code"=w462:i32)
            n198 = case shown="-314310, -314220" w462 {
              tunnel: [NetworkStreamReceiverState."Unhandled Exception" NetworkStreamReceiverState."Connection lost"] -> w461
              frame 0, Default {
              }
              frame -314310, -314220 {
                # "The remote endpoint has been destroyed."
              }
            }
          }
        }
      }
      frame "Connection lost" {
        w471 = refnum<k21> refnum  # reader endpoint
        n199 = Unbundle By Name(w472) -> ("Network Stream Reader Endpoint"=w474:refnum<k21>)
        n200 = Destroy Stream Endpoint(8:w475, 11:w474) -> (0:w469:errorcluster)
        n201 = call <vilib>:"Clear Errors.vi"("error in (no error)"=w469, "specific error code to clear (0: all)"=0) -> ("error out"=w467:errorcluster)  [unwired: 4 in, 1 out]
        n202 = Bundle By Name(cluster=w472, "Network Stream Reader Endpoint"=w471) -> (w470:T5)
      }
      frame "Exit" {
        w476 = refnum<k21> refnum  # reader endpoint
        n203 = Unbundle By Name(w481) -> ("Network Stream Reader Endpoint"=w479:refnum<k21>)
        n204 = Not Equal?(x=w476, y=w479) -> (x != y?=w478:bool)
        n205 = case shown="True" w478 {
          tunnel: w484 -> [w485 w488]
          tunnel: [w485 w487] -> w483
          tunnel: w479 -> [_ w486]
          frame False {
          }
          frame True {
            n206 = Destroy Stream Endpoint(8:w488, 11:w486) -> (0:w487:errorcluster)
          }
        }
        n207 = Bundle By Name(cluster=w481, "Network Stream Reader Endpoint"=w476) -> (w482:T5)
      }
      frame "Unhandled Exception" {
        n208 = call <vilib>:"General Error Handler.vi"("error in (no error)"=w492) -> ("error out"=w491:errorcluster)  [unwired: 10 in, 4 out]
      }
    }
    n209 = Get Queue Status(queue=w392) -> (error out=w391:errorcluster)  [unwired: 2 in, 7 out]
    n210 = case shown="Error" w391 {
      tunnel: w397 -> [w401 _]
      tunnel: [w401 NetworkStreamReceiverState."Exit"] -> w396
      frame No Error {
      }
      frame Error {
      }
    }
    "Network Stream State Indicator" <- w400
  }
  n211 = while {
    tunnel: w10 -> [w497]
    tunnel: w16 -> [w496]
    tunnel: [w495] -> w15
    tunnel: w13 -> [w494]
    tunnel: [w493] -> w12
    stop <- w498 stop-if-true
    # "Update Network Shared Status Variable"
    n212 = event shown="[1] <StatusUpdateEvent>: User Event" {
      selector: w496 -> [_ _]
      dyn-events: [_ _] -> w495
      timeout: 100 -> [_ _]
      tunnel: w494 -> [_ w508]
      tunnel: [_ w507] -> w493
      event Timeout {
        n213 = event-data() -> ()  [unwired: 1 in, 3 out]
      }
      event User Event {
        n214 = event-data() -> ("Status"=w505:string, "Data"=w503:variant, "SequenceNumber"=w502:u64)  [unwired: 1 in]
        n215 = local read "Session Hash"() -> (w504:u64)
        n216 = feedback #2() -> (w500:u64)  [unwired: 1 in]
        n217 = case shown="0" w502 {
          selector: w502 -> [w509 _]
          tunnel: [w509 w510] -> w501
          tunnel: w500 -> [_ w510]
          frame 1, Default {
          }
          frame 0 {
            # "0 as sequence number is from a command of this program. In that case just update"
          }
        }
        n218 = feedback-in #2(w501) -> ()
        n219 = Bundle("Status"=w505, "Data"=w503, "Session Hash"=w504, "SequenceNumberOfFinishedCommand"=w501) -> (w506:T11)  [unwired: 1 in]
        n220 = shared-variable "My Computer\\SolidTargetSequenceControl.lvlib\\Status"(w506, error in=w508) -> (error out=w507:errorcluster)
      }
    }
    n221 = Get Queue Status(queue=w497) -> (error out=w498:errorcluster)  [unwired: 2 in, 7 out]
  }
  n222 = Unregister For Events(event registration refnum=w15, error in=w12) -> (error out=w5:errorcluster)
  n223 = call <vilib>:"Simple Error Handler.vi"() -> ()  [unwired: 5 in, 5 out]
  n224 = Release Queue(queue=w10, error in (no error)=w8) -> (error out=w4:errorcluster)  [unwired: 1 in, 2 out]
  n225 = Merge Errors(w6, w5, w4, w3) -> (w7:errorcluster)
  n226 = disable-structure shown="RUN_TIME_ENGINE==True" {
    disable-tunnel: w7 -> [_ _]
    frame condition #0 {
      n227 = Quit LabVIEW(quit? (T)=TRUE) -> ()
    }
    frame condition #1 (active) {
    }
  }
